vi "XYZTheta Go.vi"(8 "error in (no error)":errorcluster, 10 "XYZTheta In":dbl[](array[numeric]), 11 "Motion in":refnum<class "Motion.lvclass">) -> (0 "error out":errorcluster, 2 "XYZTheta Out":dbl[](array[numeric]), 3 "Motion out":refnum<class "Motion.lvclass">)   [LabVIEW 2016, in "Motion.lvclass"]
uses:
  Motion.lvclass
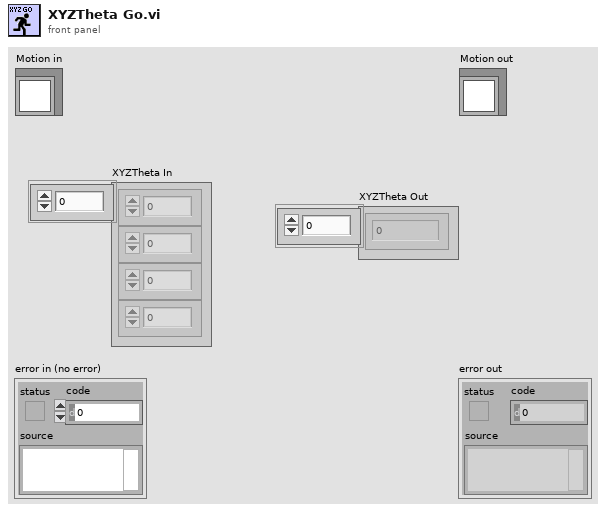
[diagram p1: front panel]
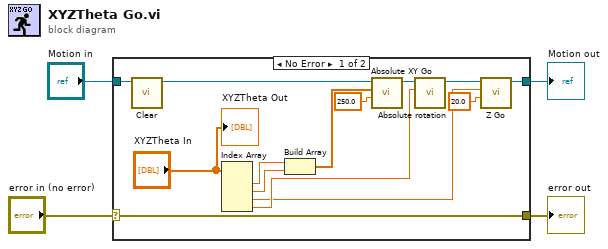
[diagram p0: block diagram]
diagram:
  n1 = case shown="No Error" "error in (no error)" {
    selector: "error in (no error)" -> [w18 w20]
    tunnel: [w18 w20] -> w1
    tunnel: [w9 w19] -> w3
    tunnel: "Motion in" -> [w17 w19]
    frame No Error {
      n2 = call "Clear.vi"("Motion in"=w17) -> ("Motion out"=w15:refnum<class "Motion.lvclass">)  [unwired: 9 in, 1 out]
      n3 = Index Array(array="XYZTheta In") -> (element #1=w6:dbl, element #2=w5:dbl, element #3=w11:dbl, element #4=w16:dbl)  [unwired: 4 in]
      n4 = Build Array(w6, w5) -> (w14:dbl[])
      n5 = call-dynamic "Absolute XY Go.vi"("Speed"=250.0, "XY"=w14, "Motion in"=w15) -> ("Motion out"=w12:refnum<class "Motion.lvclass">)  [unwired: 7 in, 1 out]
      n6 = call-dynamic "Absolute rotation.vi"("Theta"=w16, "Motion in"=w12) -> ("Motion out"=w10:refnum<class "Motion.lvclass">)  [unwired: 8 in, 1 out]
      n7 = call-dynamic "Z Go.vi"("Speed"=20.0, "Position"=w11, "Motion in"=w10) -> ("Motion out"=w9:refnum<class "Motion.lvclass">)  [unwired: 7 in, 1 out]
      "XYZTheta Out" <- "XYZTheta In"
    }
    frame Error {
    }
  }
  "error out" <- w1
  "Motion out" <- w3
